vi "Determine Funnel Points.vi"(8 "error in (no error)":errorcluster, 11 "Tool Funnel in":refnum<class "Tool Funnel.lvclass">) -> (0 "error out":errorcluster, 2 "Points":T1[](array[typedef]), 3 "Tool Funnel out":refnum<class "Tool Funnel.lvclass">)   [LabVIEW 2019, in "Tool Funnel.lvclass"]
uses:
  Tool Funnel.lvclass
  Parse/PathCommands/Point.ctl
  Parse/ParsePaths/Path.lvclass/Path.ctl
  Settings/Funnel Settings/Funnel Settings.lvclass/Funnel Settings.ctl
  Parse/PathCommands/PathCommands.lvclass
  Parse/ParsePaths/Path.lvclass
  Settings/Funnel Settings/Funnel Settings.lvclass
  Tool Path/Tool Path.lvclass
panel:
  out "XY Graph":cluster{"X":dbl, "Y":dbl}[](graph)
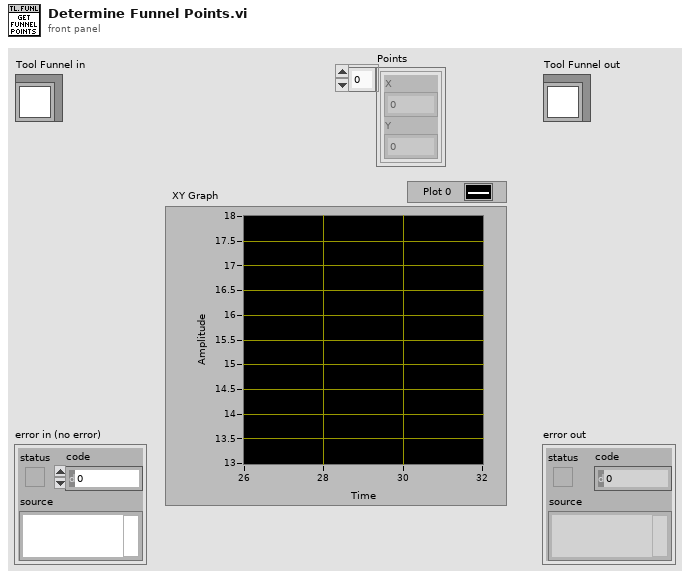
[diagram p1: front panel]
types:
  T1 = typedef "PathCommands.lvclass/Point.ctl" = cluster{"X":dbl, "Y":dbl}
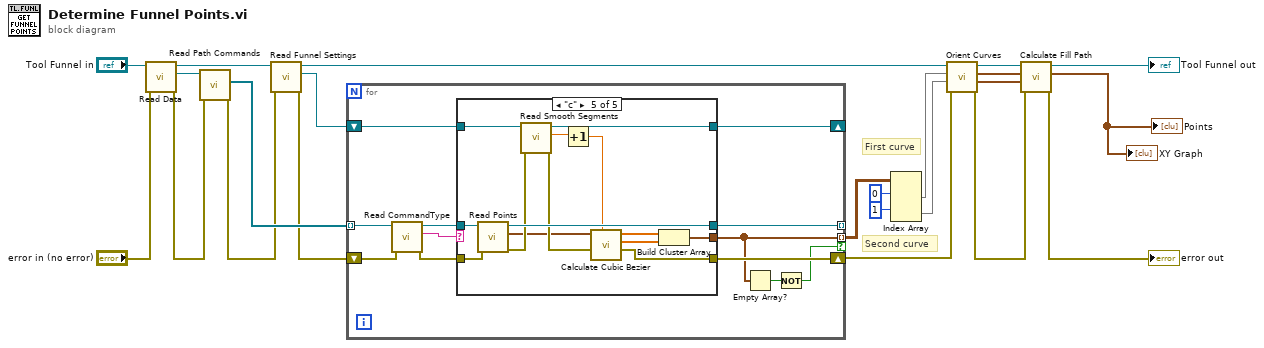
[diagram p0: block diagram]
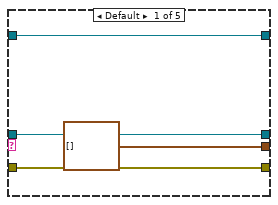
[diagram p2: hidden frame]
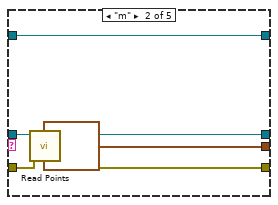
[diagram p3: hidden frame]
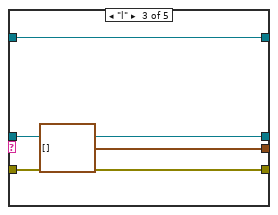
[diagram p4: hidden frame]
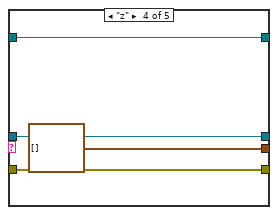
[diagram p5: hidden frame]
diagram:
  # "First curve"
  # "Second curve"
  n1 = call-dynamic "Read Data.vi"("error in (no error)"="error in (no error)", "Tool Path in"="Tool Funnel in") -> ("error out"=w21:errorcluster, "Path.lvclass"=w23:refnum<class "Path.lvclass">, "Tool Path out"=w20:refnum<class "Tool Funnel.lvclass">)  [unwired: 7 in]
  n2 = call "Read Path Commands.vi"("error in (no error)"=w21, "Path in"=w23) -> ("error out"=w8:errorcluster, "Path Commands"=w22:refnum<class "PathCommands.lvclass">[])  [unwired: 7 in, 1 out]
  n3 = call-dynamic "Read Funnel Settings.vi"("error in (no error)"=w8, "Tool Funnel in"=w20) -> ("error out"=w7:errorcluster, "Funnel Settings.lvclass"=w19:refnum<class "Funnel Settings.lvclass">, "Tool Funnel out"=w14:refnum<class "Tool Funnel.lvclass">)  [unwired: 7 in]
  n4 = for {
    shift-right: [w35] -> w6
    shift-left: w7 -> [w31]
    tunnel: w22 -> [w32] mode=indexing
    tunnel: [w34] -> _ mode=indexing
    shift-right: [w27] -> _
    shift-left: w19 -> [w28]
    tunnel: [w26] -> w5 mode=indexing if=w24
    n5 = call-dynamic "Read CommandType.vi"("error in (no error)"=w31, "PathCommands in"=w32) -> ("error out"=w30:errorcluster, "CommandType"=w29:string, "PathCommands out"=w33:refnum<class "PathCommands.lvclass">)  [unwired: 7 in]
    n6 = case shown="\"c\"" w29 {
      tunnel: [w39 w41 w47 w50 w61] -> w35
      tunnel: w30 -> [w39 w40 w47 w50 w55]
      tunnel: [w38 w44 w46 w51 w66] -> w34
      tunnel: w33 -> [w38 w45 w46 w51 w67]
      tunnel: w28 -> [w37 w43 w49 w53 w63]
      tunnel: [w37 w43 w49 w53 w64] -> w27
      tunnel: [cluster{"X":dbl, "Y":dbl}[] [] cluster{"X":dbl, "Y":dbl}[] [] cluster{"X":dbl, "Y":dbl}[] [] cluster{"X":dbl, "Y":dbl}[] [] w56] -> w26
      frame Default {
      }
      frame "m" {
        n7 = call-dynamic "Read Points.vi"("error in (no error)"=w40, "PathCommands in"=w45) -> ("error out"=w41:errorcluster, "PathCommands out"=w44:refnum<class "PathCommands.lvclass">)  [unwired: 7 in, 1 out]
      }
      frame "l" {
        # "Create interpolation VI\nCreate Distance VI"
      }
      frame "z" {
        # "Create interpolation VI\nCreate Distance VI"
      }
      frame "c" {
        n8 = call-dynamic "Read Points.vi"("error in (no error)"=w55, "PathCommands in"=w67) -> ("error out"=w65:errorcluster, "Points"=w60:T1[], "PathCommands out"=w66:refnum<class "PathCommands.lvclass">)  [unwired: 7 in]
        n9 = call "Read Smooth Segments.vi"("error in (no error)"=w65, "Funnel Settings in"=w63) -> ("error out"=w62:errorcluster, "Smooth Segments"=w59:dbl, "Funnel Settings out"=w64:refnum<class "Funnel Settings.lvclass">)  [unwired: 7 in]
        n10 = Increment(x=w59) -> (x+1=w54:dbl)
        n11 = call "Calculate Cubic Bezier.vi"("Iterations"=w54, "error in (no error)"=w62, "Points"=w60) -> ("error out"=w61:errorcluster, "Y"=w58:dbl[], "X"=w57:dbl[])  [unwired: 6 in]
        n12 = Build Cluster Array(w57, w58) -> (w56:cluster{"X":dbl, "Y":dbl}[])
      }
    }
    n13 = Empty Array?(array=w26) -> (empty?=w25:bool)
    n14 = Not(x=w25) -> (.not. x?=w24:bool)
  }
  n15 = Index Array(array=w5, index (row) #1=0 ("index (row)"), index (row) #2=1 ("index (row)")) -> (element #1=w16:cluster{"X":dbl, "Y":dbl}[], element #2=w15:cluster{"X":dbl, "Y":dbl}[])  [unwired: 2 in]
  n16 = call-dynamic "Orient Curves.vi"("error in (no error)"=w6, "Curve 2 In"=w15, "Curve 1 In"=w16, "Tool Funnel in"=w14) -> ("error out"=w11:errorcluster, "Curve 2 Out"=w12:cluster{"X":dbl, "Y":dbl}[], "Curve 1 Out"=w2:cluster{"X":dbl, "Y":dbl}[], "Tool Funnel out"=w13:refnum<class "Tool Funnel.lvclass">)  [unwired: 4 in]
  n17 = call-dynamic "Calculate Fill Path.vi"("error in (no error)"=w11, "Curve 2"=w12, "Curve 1"=w2, "Tool Funnel in"=w13) -> ("error out"=→"error out":errorcluster, "Points"=→"Points" →"XY Graph":T1[], "Tool Funnel out"=→"Tool Funnel out":refnum<class "Tool Funnel.lvclass">)  [unwired: 5 in]
